vi "horse race lamp.vi"() -> (2 "number":u32)   [LabVIEW 2014]
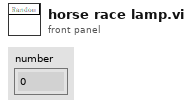
[diagram p1: front panel]
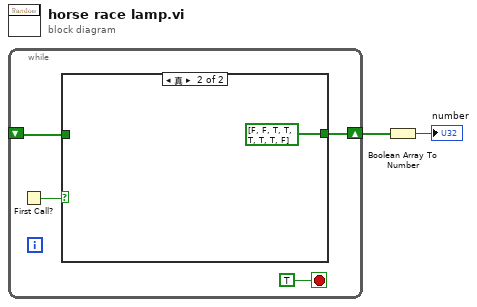
[diagram p0: block diagram]
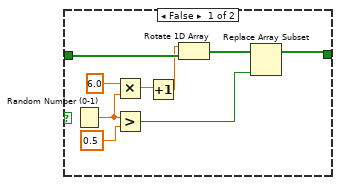
[diagram p2: hidden frame]
diagram:
  n1 = while {
    shift-right: [w5] -> w2
    shift-left: _ -> [w4]
    stop <- TRUE stop-if-true
    n2 = First Call?() -> (First Call?: T/F=w6:bool)
    n3 = case shown="真" w6 {
      tunnel: [w8 bool[] [FALSE, FALSE, TRUE, TRUE, TRUE, TRUE, TRUE, FALSE]] -> w5
      tunnel: w4 -> [w15 _]
      frame False {
        n4 = Random Number (0-1)() -> (number: 0 to 1=w7:dbl)
        n5 = Multiply(x=6.0, y=w7) -> (x*y=w10:dbl)
        n6 = Greater?(x=w7, y=0.5) -> (0:w13:bool)
        n7 = Increment(x=w10) -> (x+1=w9:dbl)
        n8 = Rotate 1D Array(1:w15, 2:w9) -> (0:w14:bool[])
        n9 = Replace Array Subset(array=w14, new element=w13) -> (w8:bool[])  [unwired: 1 in]
      }
      frame True {
      }
    }
  }
  n10 = Boolean Array To Number(Boolean array=w2) -> (number=→"number":u32)
